vi "CheckAutoLaunch.vi"(0 "error in":errorcluster, 1 "connection ID in":refnum<k5>) -> (2 "AutoLaunch?":bool, 4 "error out":errorcluster, 5 "Good Reply?":bool, 6 "ini file":string, 7 "connection ID out":refnum<k5>)   [LabVIEW 2012]
panel:
  out "Path":string
  in  "Reset":bool
  out "current state":string
  out "new file":string
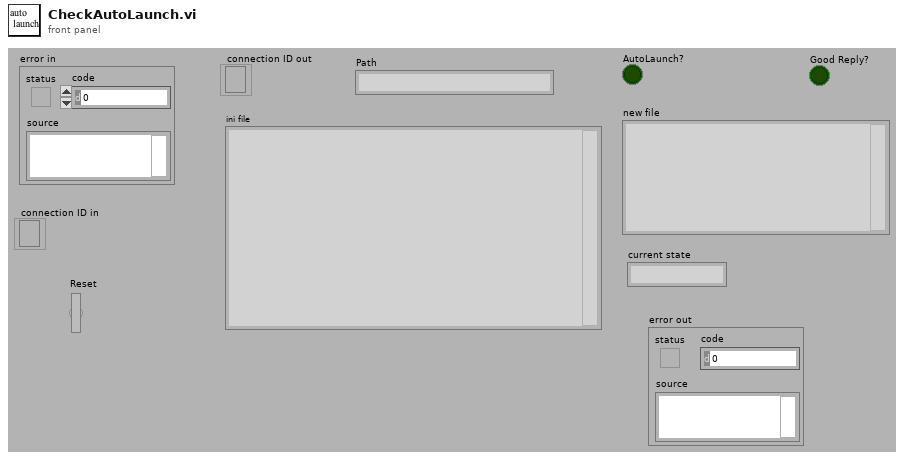
[diagram p1: front panel]
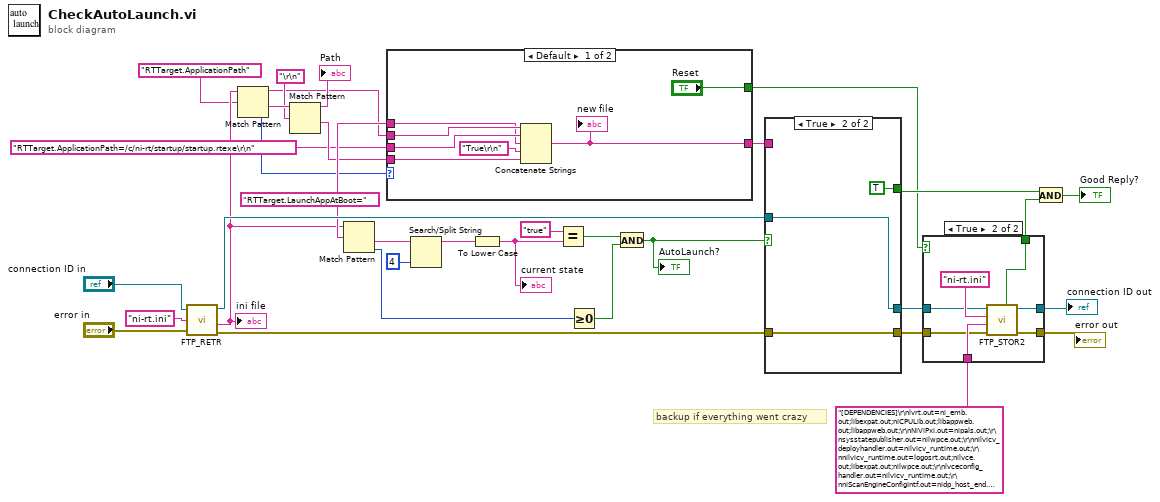
[diagram p0: block diagram]
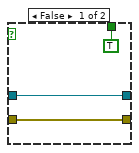
[diagram p2: hidden frame]
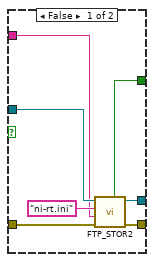
[diagram p3: hidden frame]
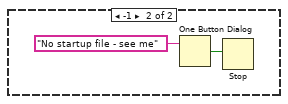
[diagram p4: hidden frame]
diagram:
  w23 = "RTTarget.LaunchAppAtBoot=" ("Remote Path")
  # "backup if everything went crazy"
  n1 = call <userlib>:"FTP_RETR.vi"("connection ID"="connection ID in", "Remote Path"="ni-rt.ini", "error in"="error in") -> ("connection ID out"=w31:refnum<k5>, "vi"=w9:string, "error out"=w33:errorcluster)  [unwired: 2 out]
  "ini file" <- w9
  n2 = Match Pattern(string=w9, regular expression="RTTarget.ApplicationPath" ("Remote Path")) -> (before substring=w4:string, after substring=w7:string, offset past match=w1:i32)  [unwired: 1 in, 1 out]
  n3 = Match Pattern(string=w7, regular expression="\r\n" ("Remote Path")) -> (before substring=→"Path":string, after substring=w3:string)  [unwired: 1 in, 2 out]
  n4 = Match Pattern(string=w9, regular expression=w23) -> (after substring=w24:string, offset past match=w22:i32)  [unwired: 1 in, 2 out]
  n5 = case shown="Default" w1 {
    tunnel: w4 -> [w41 _]
    tunnel: "RTTarget.ApplicationPath=/c/ni-rt/startup/startup.rtexe\r\n" ("Remote Path") -> [w40 _]
    tunnel: w3 -> [w38 _]
    tunnel: w23 -> [w39 _]
    tunnel: [w36 _] -> w32
    tunnel: ["Reset" _] -> w10
    frame Default {
      n6 = Concatenate Strings(w41, w40, w39, "True\r\n" ("Remote Path"), w38) -> (w36:string)
      "new file" <- w36
    }
    frame -1 {
      n7 = One Button Dialog(message="No startup file - see me") -> (true=w42:bool)  [unwired: 1 in]
      n8 = Stop(stop? (T)=w42) -> ()
    }
  }
  n9 = Search/Split String(string=w24, offset (0)=4) -> (substring before match=w26:string)  [unwired: 1 in, 2 out]
  n10 = To Lower Case(string=w26) -> (all lower case string=w27:string)
  "current state" <- w27
  n11 = Equal?(x="true", y=w27) -> (x = y?=w29:bool)
  n12 = Greater Or Equal To 0?(x=w22) -> (x >= 0?=w30:bool)
  n13 = And(x=w29, y=w30) -> (x .and. y?=w34:bool)
  "AutoLaunch?" <- w34
  n14 = case shown="True" w34 {
    tunnel: [w49 w52] -> w15
    tunnel: [w48 w53] -> w17
    tunnel: w31 -> [w47 w53]
    tunnel: w32 -> [w46 _]
    tunnel: w33 -> [w45 w52]
    tunnel: [w44 TRUE ("Good Reply?")] -> w12
    frame False {
      n15 = call <userlib>:"FTP_STOR2.vi"("error in"=w45, "File to send"=w46, "Remote Path"="ni-rt.ini" ("name or relative path"), "connection ID"=w47) -> ("Good Reply?"=w44:bool, "error out"=w49:errorcluster, "connection ID out"=w48:refnum<k5>)  [unwired: 1 in, 1 out]
    }
    frame True {
    }
  }
  n16 = case shown="True" w10 {
    tunnel: "[DEPENDENCIES]\r\nlvrt.out=ni_emb.out;libexpat.out;niCPULib.out;libappweb.out;libappweb.out;\r\nNiViPxi.out=nipals.out;\r\nsysstatepublisher.out=nilwpce.out;\r\nnilvicv_deployhandler.out=nilvicv_runtime.out;\r\nnilvicv_runtime.out=logosrt.out;nilvce.out;libexpat.out;nilwpce.out;\r\nlvceconfig_handler.out=nilvicv_runtime.out;\r\nniScanEngineConfigIntf.out=nidp_host_end.out;nilvicv_runtime.out;\r\nNiViRpc.out=nirpcs.out;\r\ncriosd.out=niriosrv.out;\r\nniriompc5125k.out=niriosrv.out;\r\nNiViSrvr.out=nirpcs.out;\r\nni_httpClient_nossl.out=nigmp.out;\r\nnisyscfg.out=nisysapi.out;\r\nniDiscExp.out=nisysapi.out;nimdnsResponder.out;niDiscSvc.out;\r\nniDiscSvc.out=nimdnsResponder.out;\r\nniorbs.out=nipals.out;nirpcs.out;\r\nnidp_target_end.out=libexpat.out;logosrt.out;\r\nnidp_host_end.out=libexpat.out;logosrt.out;\r\nvisa32.out=NiViSv32.out;\r\nNiViSys.out=nisysapi.out;visa32.out;\r\nNiFpga.out=niriosrv.out;\r\nNiRioSrv.out=libexpat.out;nirpcs.out;lvrt.out;\r\nNiRioRpc.out=NiRioSrv.out;nisvcloc.out;\r\nNiViRio.out=NiRioSrv.out;\r\nniriosae.out=nisysapi.out;niriosrv.out;\r\nNiFpgaLv.out=NiFpga.out;\r\nnisysapisvc.out=nisysrpc.out;nisysapi.out;nimdnsResponder.out;ws_runtime.out;\r\nniSysNetCfg.out=nisysapi.out;\r\nnisysrpc.out=nirpcs.out;nisysapi.out;\r\nws_runtime.out=nilwpce.out;\r\nRTWebServer.out=libappweb.out;\r\nlibniauthModule.out=nigmp.out;\r\nnilwpce.out=logosrt.out;\r\nniauth.out=nigmp.out;\r\nnipci.out=nirtdm.out;\r\n\r\n[MODULE VERSIONS]\r\nNiViEnet.out=6.3\r\nNiViPxi.out=6.3\r\nsysstatepublisher.out=6.3\r\nnilvce.out=6.3\r\nlvceconfig_handler.out=6.3\r\nnilvicv_deployhandler.out=6.3\r\nnilvicv_runtime.out=6.3\r\nniScanEngineConfigIntf.out=6.3\r\nnids.out=6.3\r\nNiEnAsrl.out=6.3\r\nNiViRpc.out=6.3\r\ncriosd.out=6.3\r\nniriompc5125k.out=6.3\r\nNiViSrvr.out=6.3\r\nnisyscfg.out=6.3\r\nniserial.out=6.3\r\nniDiscSvc.out=6.3\r\nniDiscExp.out=6.3\r\nniorbs.out=6.3\r\nnw_streams.out=6.3\r\nnidp_target_end.out=6.3\r\nnidp_host_end.out=6.3\r\nlvpidtkt.out=6.3\r\nNiViUsbj.out=6.3\r\nNILVSim.out=6.3\r\nnipals.out=6.3\r\nNiViSv32.out=6.3\r\nNiViAsrl.out=6.3\r\nvisa32.out=6.3\r\nNiViSys.out=6.3\r\nnivirio.out=6.3\r\nniriosrv.out=6.3\r\nniriorpc.out=6.3\r\nNiFpga.out=6.3\r\nNiFpgaLv.out=6.3\r\nniriosae.out=6.3\r\nnisysapisvc.out=6.3\r\nniSysNetCfg.out=6.3\r\nnisysapi.out=6.3\r\nnisysrpc.out=6.3\r\nnirpcs.out=6.3\r\nws_runtime.out=6.3\r\nnilwpce.out=6.3\r\nlogosrt.out=6.3\r\nnilxtcor.out=6.3\r\nnipspxts.out=6.3\r\nni_traceengine.out=6.3\r\nnigmp.out=6.3\r\nlvanlys.out=6.3\r\nlvblas.out=6.3\r\ngoopsup.out=6.3\r\nrendezvs.out=6.3\r\nsemaphor.out=6.3\r\nnbfifo.out=6.3\r\nsettime.out=6.3\r\nlvalarms.out=6.3\r\nlvuste.out=6.3\r\nnisvcloc.out=6.3\r\nrtvarsup.out=6.3\r\nlvrt.out=6.3\r\ntsengine.out=6.3\r\nni_emb.out=6.3\r\nvxfpsup.out=6.3\r\nnirtdm.out=6.3\r\nnipci.out=6.3\r\nlibexpat.out=6.3\r\nregistry.out=6.3\r\nftpserve.out=6.3\r\n\r\n[SUPPORTED LOCALES]\r\nchineseS=CP936\r\njapanese=CP932\r\nenglish=L1\r\n\r\n[LVRT]\r\nStartupDLLs=nisysrpc.out;NiRioRpc.out;nidp_target_end.out;niorbs.out;niserial.out;NiViSrvr.out;sysstatepublisher.out;\r\nmemoryChecking=False\r\nLABVIEWRTDir=/c/ni-rt/system\r\nPATH=/c/ni-rt/system/;/c/ni-rt/;\r\nCDIntervalTicks=55\r\nWebServer.Enabled=FALSE\r\nRTTarget.VIPath=/c/ni-rt/startup\r\nRTTarget.IPAccess=+*\r\nRTEnetRcvMode=2\r\nRTCPULoadMonitoringEnabled=True\r\nRTTarget.ApplicationPath=/c/ni-rt/startup/startup.rtexe\r\nRTTarget.LaunchAppAtBoot=True\r\nserver.tcp.access=\"+*\"\r\nRTTarget.EnableFileSharing=True\r\nserver.tcp.serviceName=\"Main Application Instance/VI Server\"\r\nRTTarget.OlsonTimeZone=\"EST\"\r\nRTTarget.TimeZone=\"EST5\"\r\n\r\n[NIDP_HANDLER_LOAD_ORDER]\r\nlvceconfig_handler.out=nilvicv_deployhandler.out;\r\n\r\n[STARTUP]\r\nEarlyStartupLibraries=nirtdm.out;nimdnsResponder.out;vxfpsup.out;tsengine.out;nisvcloc.out;RTWebServer.out;niDiscSvc.out;\r\nMainExe=/c/ni-rt/system/lvrt.out\r\nDisplayStartupLibProgress=TRUE\r\n\r\n[LOGOSXT]\r\nHeartbeat_AbsenceDetectCount=10\r\n\r\n[MDNSRESPONDER]\r\nmDNSDisableAnnouncement=0\r\nmDNSDisableDiscovery=0\r\n\r\n" ("new file 2") -> [_ w62]
    tunnel: w17 -> [w56 w61]
    tunnel: [w56 w60] -> w16
    tunnel: w15 -> [w55 w59]
    tunnel: [w55 w58] -> w14
    tunnel: [TRUE ("Good Reply?") w57] -> w13
    frame False {
    }
    frame True {
      n17 = call <userlib>:"FTP_STOR2.vi"("error in"=w59, "File to send"=w62, "Remote Path"="ni-rt.ini" ("name or relative path"), "connection ID"=w61) -> ("Good Reply?"=w57:bool, "error out"=w58:errorcluster, "connection ID out"=w60:refnum<k5>)  [unwired: 1 in, 1 out]
    }
  }
  "connection ID out" <- w16
  "error out" <- w14
  n18 = And(x=w12, y=w13) -> (x .and. y?=→"Good Reply?":bool)
